vi "ReadOrSetDefaultKeys(Int32).vi"(8 "error in (no error)":errorcluster, 9 "Default":i32[](array[numeric]), 10 "Keys":string[](array[string]), 11 "Device in":refnum<class "Device.lvclass">) -> (0 "error out":errorcluster, 2 "Values":i32[](array[numeric]), 3 "Device out":refnum<class "Device.lvclass">)   [LabVIEW 2020, in "Device.lvlib" / "Device.lvclass"]
uses:
  Device.lvclass
  Device.lvclass/Device.ctl
  <vilib>/Utility/config.llb/Read Key (I32).vi
  <vilib>/Utility/config.llb/Write Key (I32).vi
  <vilib>/Utility/config.llb/NI_LVConfig.lvlib
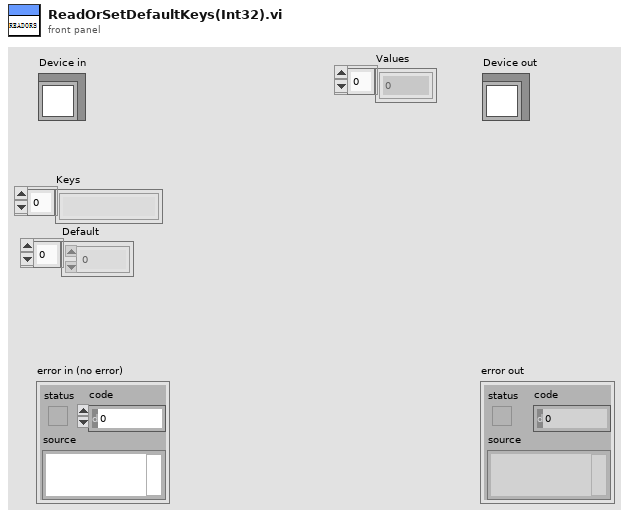
[diagram p1: front panel]
types:
  T1 = typedef "NI_LVConfig.lvlib/Config Data RefNum.ctl" = refnum<k1>
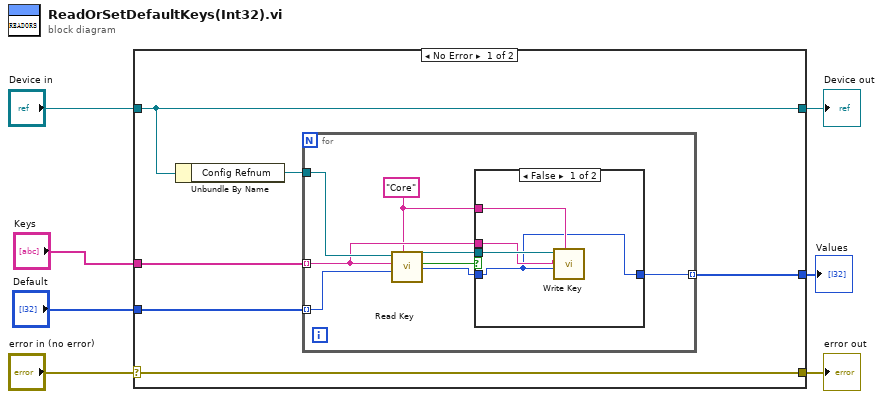
[diagram p0: block diagram]
diagram:
  n1 = case shown="No Error" "error in (no error)" {
    selector: "error in (no error)" -> [w13 w29]
    tunnel: [w13 w29] -> w6
    tunnel: [w11 w28] -> w4
    tunnel: "Device in" -> [w11 w28]
    tunnel: "Keys" -> [w12 _]
    tunnel: "Default" -> [w9 w27]
    tunnel: [w8 w27] -> w1
    frame No Error {
      n2 = Unbundle By Name(w11) -> ("Config Refnum"=w10:T1)
      n3 = for {
        tunnel: w12 -> [w17] mode=indexing
        tunnel: w10 -> [w20]
        tunnel: w9 -> [w21] mode=indexing
        tunnel: [w14] -> w8 mode=indexing
        w15 = "Core" ("section")
        n4 = call-poly <vilib>:"Read Key.vi"("section"=w15, "default value"=w21, "key"=w17, "refnum"=w20) -> ("value"=w16:i32, "found?"=w19:bool, "refnum out"=w18:T1)  [unwired: 4 in, 1 out]
        n5 = case shown="False" w19 {
          tunnel: w18 -> [w25 _]
          tunnel: w17 -> [w24 _]
          tunnel: w16 -> [w22 w26]
          tunnel: w15 -> [w23 _]
          tunnel: [w22 w26] -> w14
          frame False {
            n6 = call-poly <vilib>:"Write Key.vi"("section"=w23, "value"=w22, "key"=w24, "refnum"=w25) -> ()  [unwired: 5 in, 3 out]
          }
          frame True {
          }
        }
      }
    }
    frame Error {
    }
  }
  "error out" <- w6
  "Device out" <- w4
  "Values" <- w1
